vi "Negate (multiple).vi"(8 "error in (no error)":errorcluster, 11 "XY-data":cluster{"X-array":dbl[], "Y-array":dbl[]}[](array[cluster]) {"Y-array" format="%.2p"; "X-array" format="%.2p"}) -> (0 "error out":errorcluster, 3 "XY-data out":cluster{"X-array":dbl[], "Y-array":dbl[]}[](array[cluster]) {"Y-array" format="%.2p"; "X-array" format="%.2p"})   [LabVIEW 2019, in "xy_utilities.lvlib"]
doc: "Negates <b>XY-data</b>'s y array.\n\nWire data to the data input to determine the polymorphic instance to use or manually select the instance."
uses:
  xy_utilities.lvlib
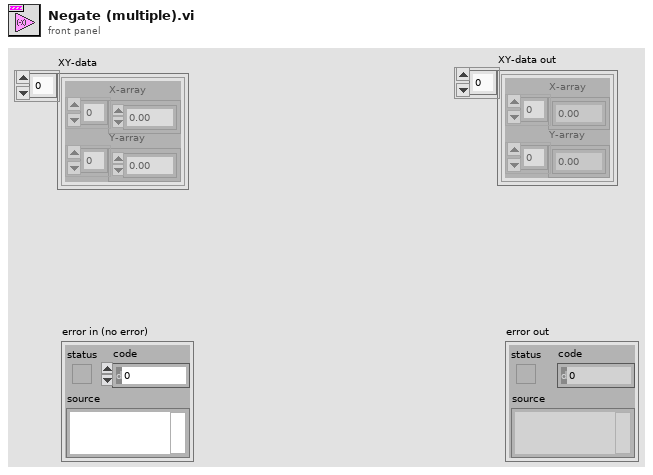
[diagram p1: front panel]
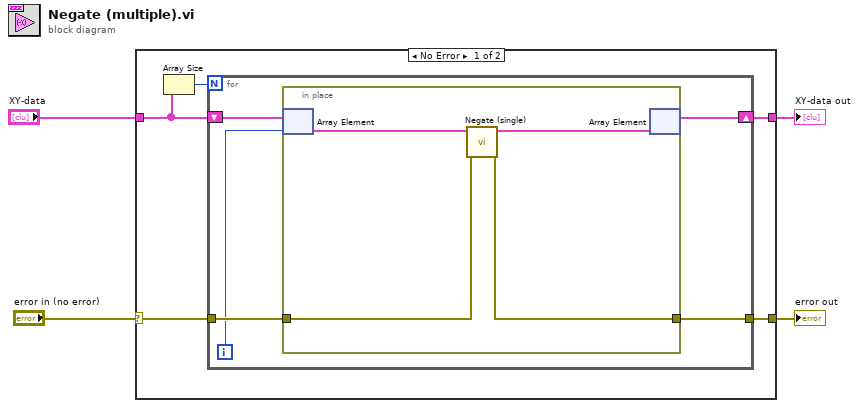
[diagram p0: block diagram]
diagram:
  n1 = case shown="No Error" "error in (no error)" {
    selector: "error in (no error)" -> [w8 w20]
    tunnel: [w7 w20] -> w3
    tunnel: "XY-data" -> [w5 w19]
    tunnel: [w9 w19] -> w1
    frame No Error {
      n2 = Array Size(array=w5) -> (size(s)=w6:i32)
      n3 = for {
        N: w6 -> [_]
        tunnel: w8 -> [w14]
        tunnel: [w13] -> w7
        shift-right: [w10] -> w9
        shift-left: w5 -> [w12]
        i -> [w11]
        n4 = in-place {
          in-place-border: w14 -> [w18]
          in-place-border: [w17] -> w13
          n5 = in-place-array #1(w12, w11) -> (w16:cluster{"X-array":dbl[], "Y-array":dbl[]})
          n6 = call "Negate (single).vi"("error in (no error)"=w18, "XY-data"=w16) -> ("error out"=w17:errorcluster, "XY-data out"=w15:cluster{"X-array":dbl[], "Y-array":dbl[]})  [unwired: 8 in]
          n7 = in-place-array #1(w15) -> (w10:cluster{"X-array":dbl[], "Y-array":dbl[]}[])  [unwired: 1 out]
        }
      }
    }
    frame Error {
    }
  }
  "error out" <- w3
  "XY-data out" <- w1
